vi "PYTHON Set Server Path__ogtk.vi"(4 "error in (no error)":errorcluster, 6 "token (empty: \"PythonServer\")":string, 7 "path (empty: python24.dll)":path) -> (0 "error out":errorcluster)   [LabVIEW 2012]
doc: "This function configures the interface to use a particular Python shared library."
uses:
  <userlib>/_OpenG.lib/labpython/lvpython.dll
panel:
  # "possible values : PythonServer\n                           ArrayModule"
  # "PYTHON Set Server Path.vi\n\nConfigures the interface to use a particular Python shared library\n\nCopyright (C) 2002 Rolf Kalbermatter rolf.kalbermatter@citeng.com\nCopyright (C) 2002 James Kring jim@jimkring.com\n\nPlease visit http://www.OpenG.org to learn about the\nOpen Source LabVIEW software movement.\n\nThis library is free software; you can redistribute it and/or\nmodify it under the terms of the GNU Lesser General Public\nLicense as published by the Free Software Foundation; either\nversion 2.1 of the License, or (at your option) any later version.\nThis library is distributed in the hope that it will be useful,\nbut WITHOUT ANY WARRANTY; without even the implied warranty of\nMERCHANTABILITY or FITNESS FOR A PARTICULAR PURPOSE. See the GNU\nLesser General Public License for more details.\nYou should have received a copy of the GNU Lesser General Public\nLicense along with this library; if not, write to the Free Software\nFoundation, Inc., 59 Temple Place, Suite 330, Boston, MA 02111-1307 USA"
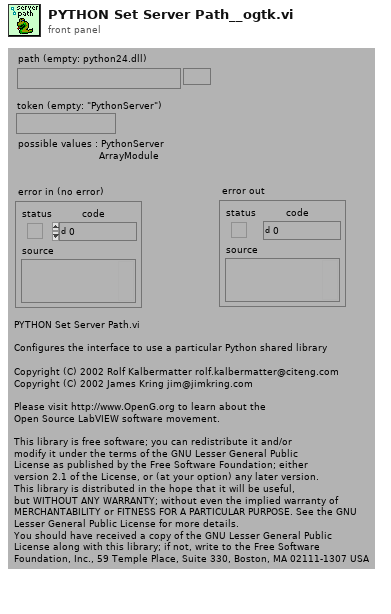
[diagram p1: front panel]
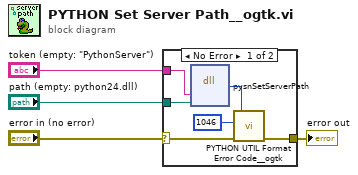
[diagram p0: block diagram]
diagram:
  n1 = case shown="No Error" "error in (no error)" {
    selector: "error in (no error)" -> [w10 w11]
    tunnel: [w9 w11] -> w3
    tunnel: "path (empty: python24.dll)" -> [w6 _]
    tunnel: "token (empty: \"PythonServer\")" -> [w5 _]
    frame No Error {
      n2 = dll-call lib="C:/Program Files/National Instruments/LabVIEW 2012/user.lib/_OpenG.lib/labpython/lvpython.*" fn="pysnSetServerPath"("token"=w5, "path (empty: python24.dll)"=w6) -> (w7:i32)  [unwired: 5 in, 2 out]
      n3 = call <userlib>:"PYTHON UTIL Format Error Code__ogtk.vi"("error in (no error)"=w10, "code"=1046, "Bool32"=w7) -> ("error out"=w9:errorcluster)  [unwired: 4 in]
    }
    frame Error {
    }
  }
  "error out" <- w3
